vi "条件探针，队列.vi"   [LabVIEW 2021]
doc: "本VI是为《我和LabVIEW》一书编写的示例。\n关于本书的介绍请参考网页：\nhttp://ruanqizhen.spaces.live.com/blog/cns!5852D4F797C53FB6!4310.entry"
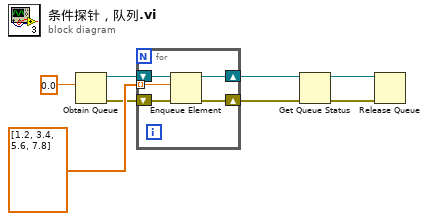
[diagram p0: block diagram]
diagram:
  n1 = Obtain Queue(element data type=0.0) -> (queue out=w8:refnum<queue>, error out=w5:errorcluster)  [unwired: 3 in, 2 out]
  n2 = for {
    tunnel: dbl[] [1.2, 3.4, 5.6, 7.8] -> [w12] mode=indexing
    shift-right: [w10] -> w3
    shift-left: w5 -> [w11]
    shift-right: [w9] -> w4
    shift-left: w8 -> [w13]
    n3 = Enqueue Element(queue=w13, element=w12, error in (no error)=w11) -> (queue out=w9:refnum<queue>, error out=w10:errorcluster)  [unwired: 2 out]
  }
  n4 = Get Queue Status(queue=w4, error in (no error)=w3) -> (queue out=w2:refnum<queue>, error out=w1:errorcluster)  [unwired: 7 out]
  n5 = Release Queue(queue=w2, error in (no error)=w1) -> ()  [unwired: 4 out]
